vi "КЛАВИАТУРА ПОЛНАЯSMALL.vi"(8 "ВХОД ИЗМЕНЕНИЕ":string, 11 "ВХОД СТАРОЕ":string) -> (3 "ВЫХОД РЕЗУЛЬТАТ":string)   [LabVIEW 2016, in "Library.lvlib"]
uses:
  Granule-2000AT/PC/Library.lvlib
panel:
  in  "+":bool
  in  "УДАЛИТЬ":bool
  in  "ОТМЕНА":bool
  in  "ВВОД":bool
  in  "0":bool
  in  "3":bool
  in  "2":bool
  in  "1":bool
  in  "6":bool
  in  "5":bool
  in  "4":bool
  in  "8":bool
  in  "9":bool
  in  "7":bool
  in  "ПРОБЕЛ":bool
  in  "/":bool
  in  "Ю":bool
  in  "Б":bool
  in  "Ь":bool
  in  "Т":bool
  in  "И":bool
  in  "М":bool
  in  "С":bool
  in  "Ч":bool
  in  "Я":bool
  in  "\\":bool
  in  "Э":bool
  in  "Ж":bool
  in  "Д":bool
  in  "Л":bool
  in  "О":bool
  in  "Р":bool
  in  "П":bool
  in  "А":bool
  in  "В":bool
  in  "Ы":bool
  in  "Ф":bool
  in  "Ъ":bool
  in  "Х":bool
  in  "З":bool
  in  "Щ":bool
  in  "Ш":bool
  in  "Г":bool
  in  "Н":bool
  in  "Е":bool
  in  "К":bool
  in  "У":bool
  in  "Ц":bool
  in  "Й":bool
  in  "-":bool
  in  "RU":bool
  in  "=":bool
  in  ")":bool
  in  "(":bool
  in  "*":bool
  in  "?":bool
  in  ":":bool
  in  "%":bool
  in  ";":bool
  in  "№":bool
  in  "\"":bool
  in  "!":bool
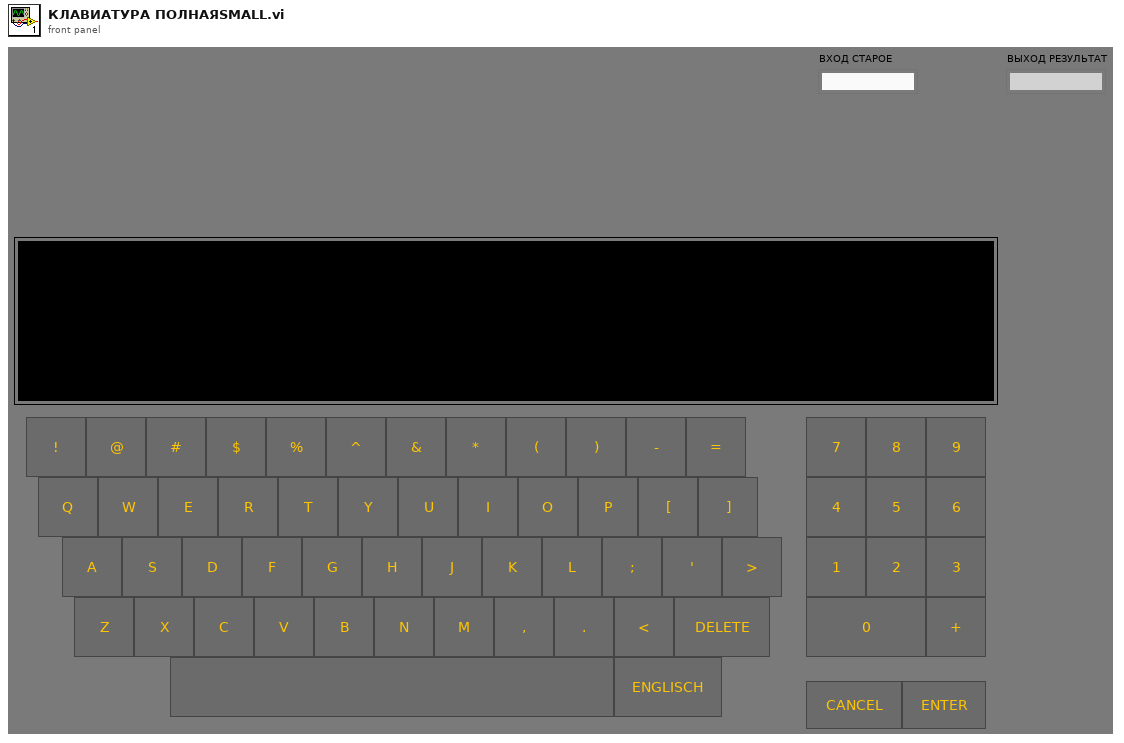
[diagram p1: front panel]
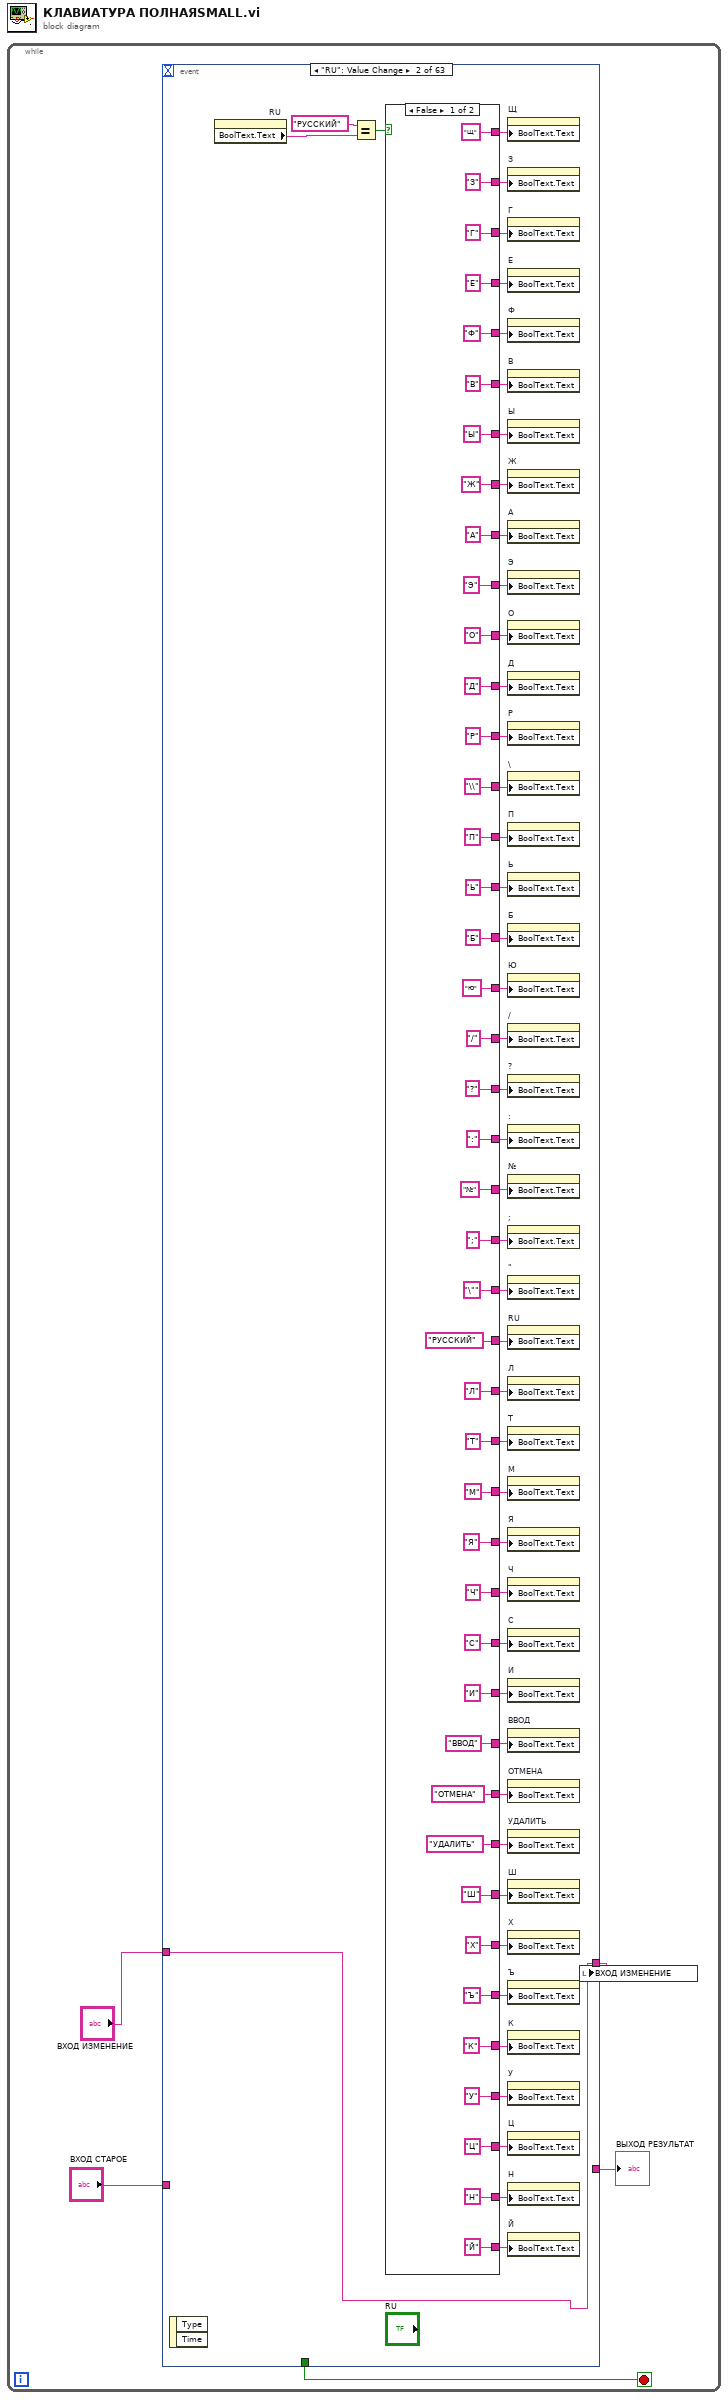
[diagram p0: block diagram]
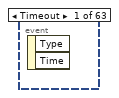
[diagram p2: hidden frame]
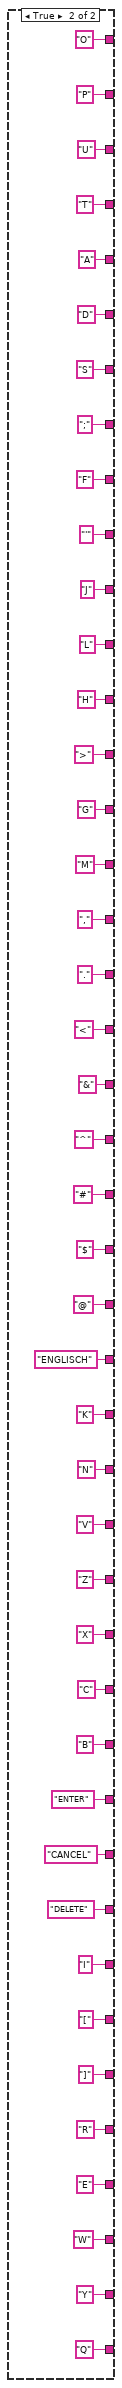
[diagram p3: hidden frame]
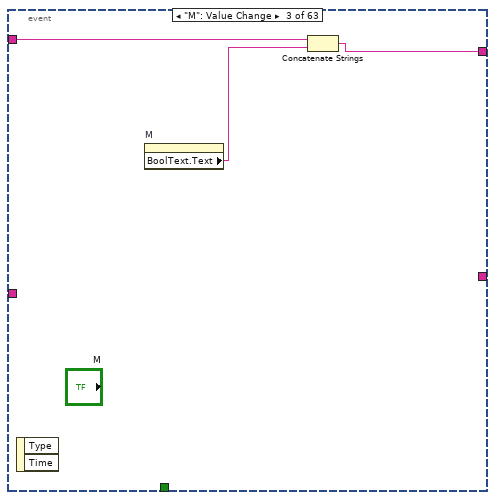
[diagram p4: hidden frame]
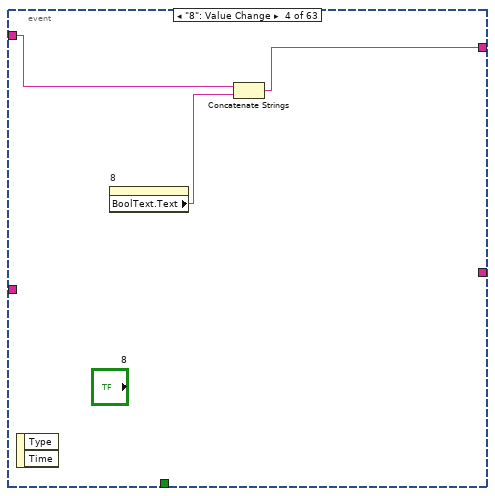
[diagram p5: hidden frame]
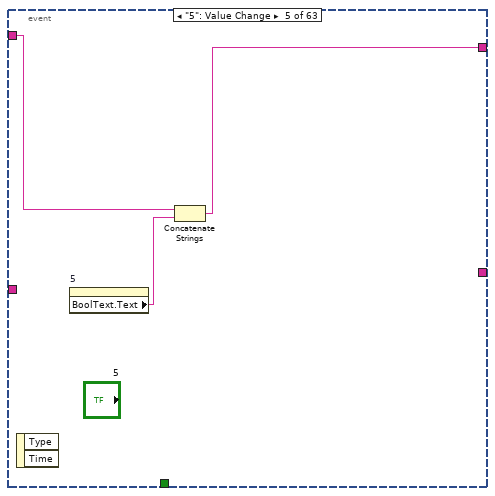
[diagram p6: hidden frame]
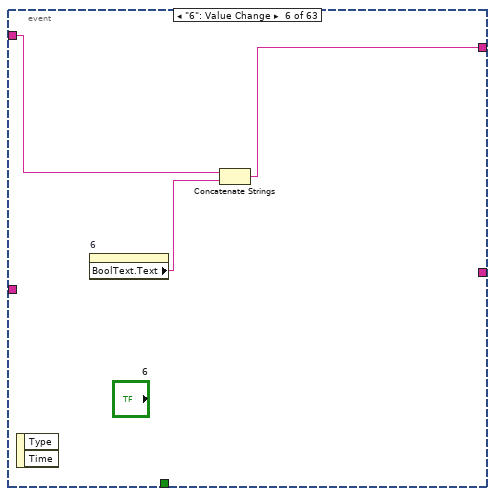
[diagram p7: hidden frame]
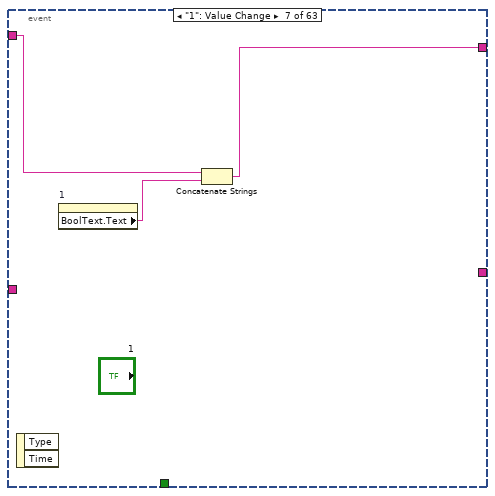
[diagram p8: hidden frame]
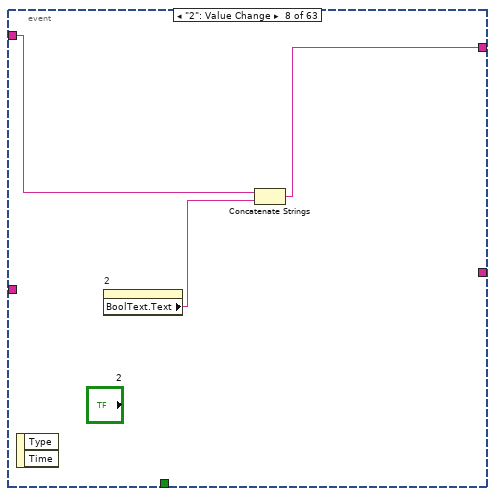
[diagram p9: hidden frame]
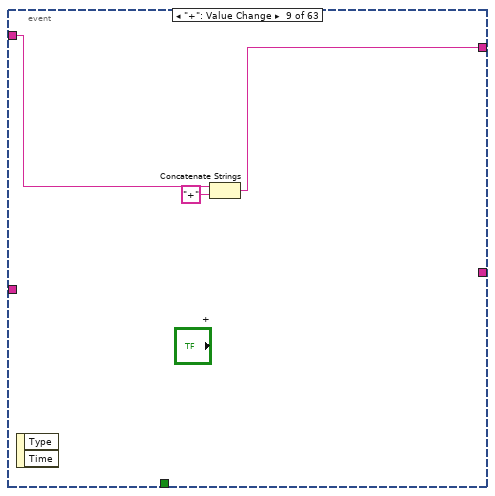
[diagram p10: hidden frame]
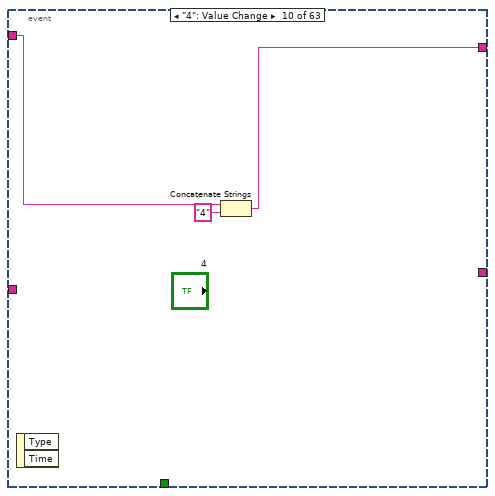
[diagram p11: hidden frame]
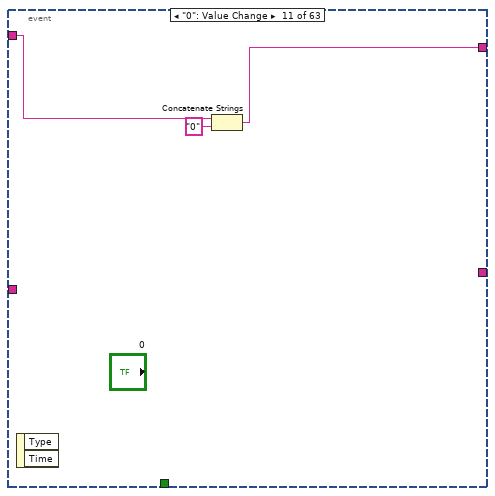
[diagram p12: hidden frame]
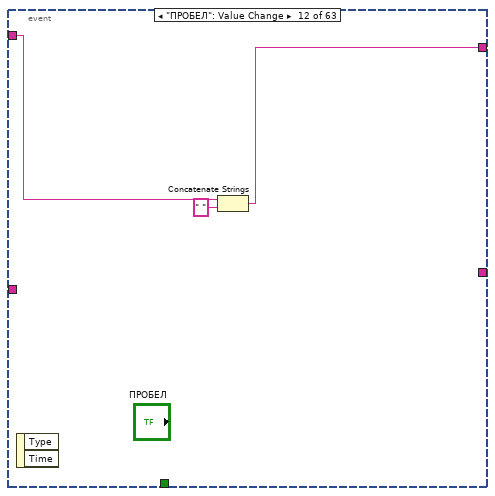
[diagram p13: hidden frame]
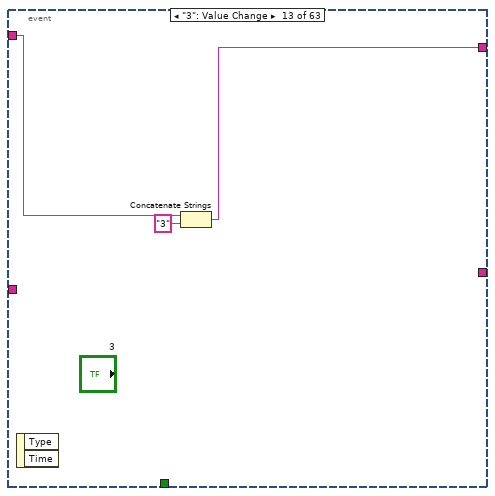
[diagram p14: hidden frame]
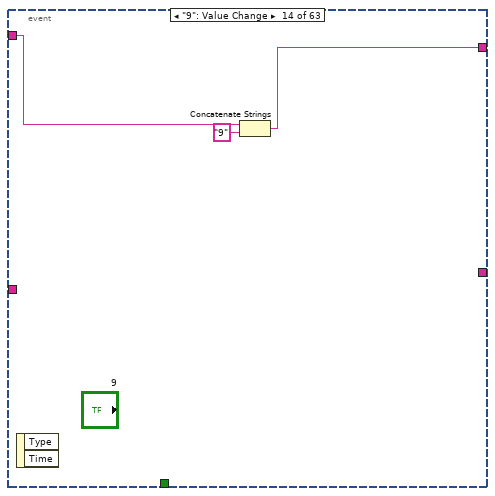
[diagram p15: hidden frame]
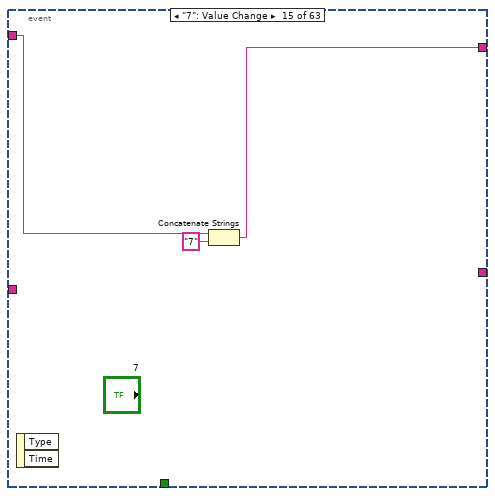
[diagram p16: hidden frame]
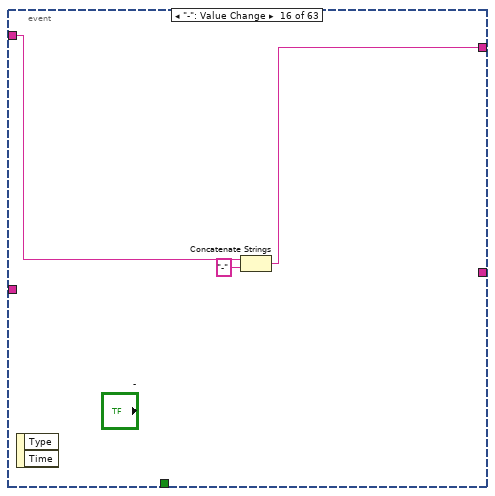
[diagram p17: hidden frame]
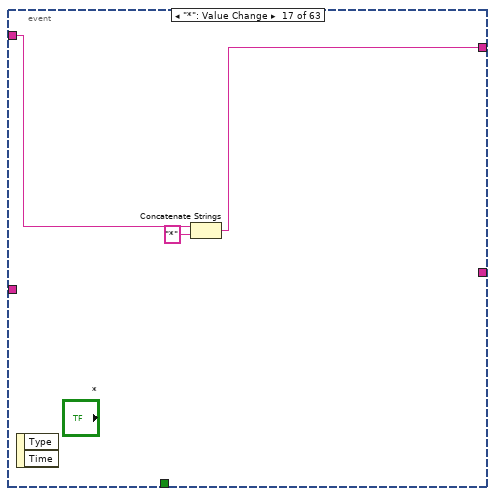
[diagram p18: hidden frame]
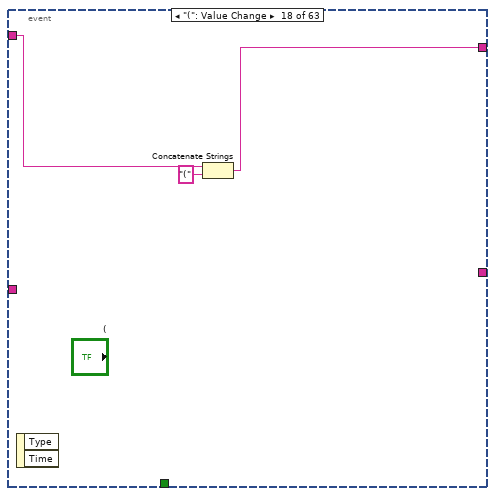
[diagram p19: hidden frame]
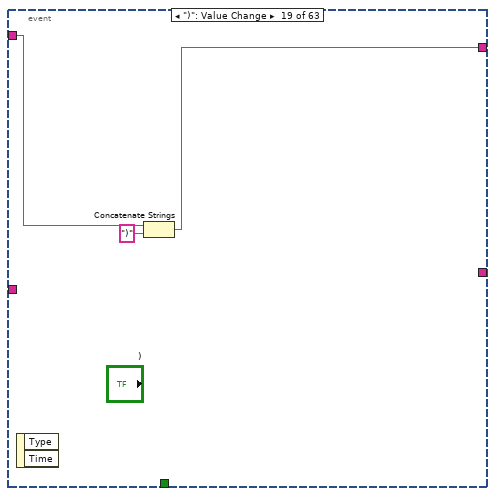
[diagram p20: hidden frame]
diagram:
  n1 = while {
    stop <- w1 stop-if-true
    n2 = event shown="[1] \"RU\": Value Change" {
      selector: _ -> [_ _ _ _ _ _ _ _ _ _ _ _ _ _ _ _ _ _ _ _ _ _ _ _ _ _ _ _ _ _ _ _ _ _ _ _ _ _ _ _ _ _ _ _ _ _ _ _ _ _ _ _ _ _ _ _ _ _ _ _ _ _ _]
      dyn-events: _ -> [_ _ _ _ _ _ _ _ _ _ _ _ _ _ _ _ _ _ _ _ _ _ _ _ _ _ _ _ _ _ _ _ _ _ _ _ _ _ _ _ _ _ _ _ _ _ _ _ _ _ _ _ _ _ _ _ _ _ _ _ _ _ _]
      timeout: _ -> [_ _ _ _ _ _ _ _ _ _ _ _ _ _ _ _ _ _ _ _ _ _ _ _ _ _ _ _ _ _ _ _ _ _ _ _ _ _ _ _ _ _ _ _ _ _ _ _ _ _ _ _ _ _ _ _ _ _ _ _ _ _ _]
      tunnel: "ВХОД ИЗМЕНЕНИЕ" -> [_ w6 w141 w144 w147 w149 w153 w156 w159 w162 w165 w168 w171 w174 w177 w180 w183 w186 w189 w192 w199 w205 w207 w211 w214 w217 w219 w222 w225 w229 w232 w234 w238 w240 w244 w246 w249 w252 w256 w258 w262 w265 w268 w270 w273 w277 w280 w283 w286 w289 w292 w295 w297 w300 w304 w307 w310 w313 w315 w318 w322 w323 w327]
      tunnel: [_ w6 w139 w143 w146 w148 w151 w155 w157 w160 w163 w167 w169 w172 w175 w178 w181 w184 w188 w190 w198 w203 w206 w209 w212 w215 w218 w221 w224 w227 w230 w233 w236 w239 w243 w245 w248 w251 w254 w257 w260 w264 w266 w269 w272 w275 w278 w281 w284 w287 w290 w293 w296 w299 w302 w305 w308 w311 w314 w317 w321 w323 w327] -> w4
      tunnel: [_ _ _ _ _ _ _ _ _ _ _ _ _ _ _ _ _ _ _ _ _ _ _ _ _ _ _ _ _ _ _ _ _ _ _ _ _ _ _ _ _ _ _ _ _ _ _ _ _ _ _ _ _ _ _ _ _ _ _ _ _ w325 w327] -> w3
      tunnel: "ВХОД СТАРОЕ" -> [_ _ _ _ _ _ _ _ _ _ _ _ _ _ _ _ _ _ _ _ _ _ _ _ _ _ _ _ _ _ _ _ _ _ _ _ _ _ _ _ _ _ _ _ _ _ _ _ _ _ _ _ _ _ _ _ _ _ _ _ _ w325 _]
      tunnel: [_ _ _ _ _ _ _ _ _ _ _ _ _ _ _ _ _ _ _ _ _ _ _ _ _ _ _ _ _ _ _ _ _ _ _ _ _ _ _ _ _ _ _ _ _ _ _ _ _ _ _ _ _ _ _ _ _ _ _ _ _ "ОТМЕНА" "ВВОД"] -> w1
      event Timeout {
        n3 = event-data() -> ()  [unwired: 1 in, 2 out]
      }
      event "RU": Value Change {
        n4 = event-data() -> ()  [unwired: 1 in, 2 out]
        n5 = property on="RU" class="Bool"() -> ("BoolText.Text"=w51:string)  [unwired: 2 in, 2 out]
        n6 = Equal?(x="РУССКИЙ", y=w51) -> (x = y?=w52:bool)
        n7 = case shown="False" w52 {
          tunnel: ["РУССКИЙ" ("Boolean Text.Text") "ENGLISCH" ("Boolean Text.Text")] -> w49
          tunnel: ["\"" ("Boolean Text.Text") "@" ("Boolean Text.Text")] -> w48
          tunnel: [";" ("Boolean Text.Text") "$" ("Boolean Text.Text")] -> w47
          tunnel: ["№" ("Boolean Text.Text") "#" ("Boolean Text.Text")] -> w46
          tunnel: [":" ("Boolean Text.Text") "^" ("Boolean Text.Text")] -> w45
          tunnel: ["?" ("Boolean Text.Text") "&" ("Boolean Text.Text")] -> w44
          tunnel: ["Й" ("Boolean Text.Text") "Q" ("Boolean Text.Text")] -> w43
          tunnel: ["Н" ("Boolean Text.Text") "Y" ("Boolean Text.Text")] -> w42
          tunnel: ["Ц" ("Boolean Text.Text") "W" ("Boolean Text.Text")] -> w41
          tunnel: ["У" ("Boolean Text.Text") "E" ("Boolean Text.Text")] -> w40
          tunnel: ["К" ("Boolean Text.Text") "R" ("Boolean Text.Text")] -> w39
          tunnel: ["Ъ" ("Boolean Text.Text") "]" ("Boolean Text.Text")] -> w38
          tunnel: ["Х" ("Boolean Text.Text") "[" ("Boolean Text.Text")] -> w37
          tunnel: ["Ш" ("Boolean Text.Text") "I" ("Boolean Text.Text")] -> w36
          tunnel: ["Щ" ("Boolean Text.Text") "O" ("Boolean Text.Text")] -> w35
          tunnel: ["З" ("Boolean Text.Text") "P" ("Boolean Text.Text")] -> w34
          tunnel: ["Г" ("Boolean Text.Text") "U" ("Boolean Text.Text")] -> w33
          tunnel: ["Е" ("Boolean Text.Text") "T" ("Boolean Text.Text")] -> w32
          tunnel: ["Ф" ("Boolean Text.Text") "A" ("Boolean Text.Text")] -> w31
          tunnel: ["В" ("Boolean Text.Text") "D" ("Boolean Text.Text")] -> w30
          tunnel: ["Ы" ("Boolean Text.Text") "S" ("Boolean Text.Text")] -> w29
          tunnel: ["Ж" ("Boolean Text.Text") ";" ("Boolean Text.Text")] -> w28
          tunnel: ["А" ("Boolean Text.Text") "F" ("Boolean Text.Text")] -> w27
          tunnel: ["Э" ("Boolean Text.Text") "'" ("Boolean Text.Text")] -> w26
          tunnel: ["О" ("Boolean Text.Text") "J" ("Boolean Text.Text")] -> w25
          tunnel: ["Д" ("Boolean Text.Text") "L" ("Boolean Text.Text")] -> w24
          tunnel: ["Р" ("Boolean Text.Text") "H" ("Boolean Text.Text")] -> w23
          tunnel: ["\\" ("Boolean Text.Text") ">" ("Boolean Text.Text")] -> w22
          tunnel: ["П" ("Boolean Text.Text") "G" ("Boolean Text.Text")] -> w21
          tunnel: ["Л" ("Boolean Text.Text") "K" ("Boolean Text.Text")] -> w20
          tunnel: ["ОТМЕНА" ("Boolean Text.Text") "CANCEL" ("Boolean Text.Text")] -> w19
          tunnel: ["ВВОД" ("Boolean Text.Text") "ENTER" ("Boolean Text.Text")] -> w18
          tunnel: ["УДАЛИТЬ" ("Boolean Text.Text") "DELETE" ("Boolean Text.Text")] -> w17
          tunnel: ["Я" ("Boolean Text.Text") "Z" ("Boolean Text.Text")] -> w16
          tunnel: ["Ч" ("Boolean Text.Text") "X" ("Boolean Text.Text")] -> w15
          tunnel: ["С" ("Boolean Text.Text") "C" ("Boolean Text.Text")] -> w14
          tunnel: ["М" ("Boolean Text.Text") "V" ("Boolean Text.Text")] -> w13
          tunnel: ["И" ("Boolean Text.Text") "B" ("Boolean Text.Text")] -> w12
          tunnel: ["Т" ("Boolean Text.Text") "N" ("Boolean Text.Text")] -> w11
          tunnel: ["Ь" ("Boolean Text.Text") "M" ("Boolean Text.Text")] -> w10
          tunnel: ["Б" ("Boolean Text.Text") "," ("Boolean Text.Text")] -> w9
          tunnel: ["Ю" ("Boolean Text.Text") "." ("Boolean Text.Text")] -> w8
          tunnel: ["/" ("Boolean Text.Text") "<" ("Boolean Text.Text")] -> w7
          frame False {
          }
          frame True {
          }
        }
        n8 = property on="Щ" class="Bool"("BoolText.Text"=w35) -> ()  [unwired: 2 in, 2 out]
        n9 = property on="З" class="Bool"("BoolText.Text"=w34) -> ()  [unwired: 2 in, 2 out]
        n10 = property on="Г" class="Bool"("BoolText.Text"=w33) -> ()  [unwired: 2 in, 2 out]
        n11 = property on="Е" class="Bool"("BoolText.Text"=w32) -> ()  [unwired: 2 in, 2 out]
        n12 = property on="Ф" class="Bool"("BoolText.Text"=w31) -> ()  [unwired: 2 in, 2 out]
        n13 = property on="В" class="Bool"("BoolText.Text"=w30) -> ()  [unwired: 2 in, 2 out]
        n14 = property on="Ы" class="Bool"("BoolText.Text"=w29) -> ()  [unwired: 2 in, 2 out]
        n15 = property on="Ж" class="Bool"("BoolText.Text"=w28) -> ()  [unwired: 2 in, 2 out]
        n16 = property on="А" class="Bool"("BoolText.Text"=w27) -> ()  [unwired: 2 in, 2 out]
        n17 = property on="Э" class="Bool"("BoolText.Text"=w26) -> ()  [unwired: 2 in, 2 out]
        n18 = property on="О" class="Bool"("BoolText.Text"=w25) -> ()  [unwired: 2 in, 2 out]
        n19 = property on="Д" class="Bool"("BoolText.Text"=w24) -> ()  [unwired: 2 in, 2 out]
        n20 = property on="Р" class="Bool"("BoolText.Text"=w23) -> ()  [unwired: 2 in, 2 out]
        n21 = property on="\\" class="Bool"("BoolText.Text"=w22) -> ()  [unwired: 2 in, 2 out]
        n22 = property on="П" class="Bool"("BoolText.Text"=w21) -> ()  [unwired: 2 in, 2 out]
        n23 = property on="Ь" class="Bool"("BoolText.Text"=w10) -> ()  [unwired: 2 in, 2 out]
        n24 = property on="Б" class="Bool"("BoolText.Text"=w9) -> ()  [unwired: 2 in, 2 out]
        n25 = property on="Ю" class="Bool"("BoolText.Text"=w8) -> ()  [unwired: 2 in, 2 out]
        n26 = property on="/" class="Bool"("BoolText.Text"=w7) -> ()  [unwired: 2 in, 2 out]
        n27 = property on="?" class="Bool"("BoolText.Text"=w44) -> ()  [unwired: 2 in, 2 out]
        n28 = property on=":" class="Bool"("BoolText.Text"=w45) -> ()  [unwired: 2 in, 2 out]
        n29 = property on="№" class="Bool"("BoolText.Text"=w46) -> ()  [unwired: 2 in, 2 out]
        n30 = property on=";" class="Bool"("BoolText.Text"=w47) -> ()  [unwired: 2 in, 2 out]
        n31 = property on="\"" class="Bool"("BoolText.Text"=w48) -> ()  [unwired: 2 in, 2 out]
        n32 = property on="RU" class="Bool"("BoolText.Text"=w49) -> ()  [unwired: 2 in, 2 out]
        n33 = property on="Л" class="Bool"("BoolText.Text"=w20) -> ()  [unwired: 2 in, 2 out]
        n34 = property on="Т" class="Bool"("BoolText.Text"=w11) -> ()  [unwired: 2 in, 2 out]
        n35 = property on="М" class="Bool"("BoolText.Text"=w13) -> ()  [unwired: 2 in, 2 out]
        n36 = property on="Я" class="Bool"("BoolText.Text"=w16) -> ()  [unwired: 2 in, 2 out]
        n37 = property on="Ч" class="Bool"("BoolText.Text"=w15) -> ()  [unwired: 2 in, 2 out]
        n38 = property on="С" class="Bool"("BoolText.Text"=w14) -> ()  [unwired: 2 in, 2 out]
        n39 = property on="И" class="Bool"("BoolText.Text"=w12) -> ()  [unwired: 2 in, 2 out]
        n40 = property on="ВВОД" class="Bool"("BoolText.Text"=w18) -> ()  [unwired: 2 in, 2 out]
        n41 = property on="ОТМЕНА" class="Bool"("BoolText.Text"=w19) -> ()  [unwired: 2 in, 2 out]
        n42 = property on="УДАЛИТЬ" class="Bool"("BoolText.Text"=w17) -> ()  [unwired: 2 in, 2 out]
        n43 = property on="Ш" class="Bool"("BoolText.Text"=w36) -> ()  [unwired: 2 in, 2 out]
        n44 = property on="Х" class="Bool"("BoolText.Text"=w37) -> ()  [unwired: 2 in, 2 out]
        n45 = property on="Ъ" class="Bool"("BoolText.Text"=w38) -> ()  [unwired: 2 in, 2 out]
        n46 = property on="К" class="Bool"("BoolText.Text"=w39) -> ()  [unwired: 2 in, 2 out]
        n47 = property on="У" class="Bool"("BoolText.Text"=w40) -> ()  [unwired: 2 in, 2 out]
        n48 = property on="Ц" class="Bool"("BoolText.Text"=w41) -> ()  [unwired: 2 in, 2 out]
        n49 = property on="Н" class="Bool"("BoolText.Text"=w42) -> ()  [unwired: 2 in, 2 out]
        n50 = property on="Й" class="Bool"("BoolText.Text"=w43) -> ()  [unwired: 2 in, 2 out]
      }
      event "М": Value Change {
        n51 = event-data() -> ()  [unwired: 1 in, 2 out]
        n52 = property on="М" class="Bool"() -> ("BoolText.Text"=w140:string)  [unwired: 2 in, 2 out]
        n53 = Concatenate Strings(w141, w140) -> (w139:string)
      }
      event "8": Value Change {
        n54 = event-data() -> ()  [unwired: 1 in, 2 out]
        n55 = property on="8" class="Bool"() -> ("BoolText.Text"=w142:string)  [unwired: 2 in, 2 out]
        n56 = Concatenate Strings(w144, w142) -> (w143:string)
      }
      event "5": Value Change {
        n57 = event-data() -> ()  [unwired: 1 in, 2 out]
        n58 = property on="5" class="Bool"() -> ("BoolText.Text"=w145:string)  [unwired: 2 in, 2 out]
        n59 = Concatenate Strings(w147, w145) -> (w146:string)
      }
      event "6": Value Change {
        n60 = event-data() -> ()  [unwired: 1 in, 2 out]
        n61 = property on="6" class="Bool"() -> ("BoolText.Text"=w150:string)  [unwired: 2 in, 2 out]
        n62 = Concatenate Strings(w149, w150) -> (w148:string)
      }
      event "1": Value Change {
        n63 = event-data() -> ()  [unwired: 1 in, 2 out]
        n64 = property on="1" class="Bool"() -> ("BoolText.Text"=w152:string)  [unwired: 2 in, 2 out]
        n65 = Concatenate Strings(w153, w152) -> (w151:string)
      }
      event "2": Value Change {
        n66 = event-data() -> ()  [unwired: 1 in, 2 out]
        n67 = property on="2" class="Bool"() -> ("BoolText.Text"=w154:string)  [unwired: 2 in, 2 out]
        n68 = Concatenate Strings(w156, w154) -> (w155:string)
      }
      event "+": Value Change {
        n69 = event-data() -> ()  [unwired: 1 in, 2 out]
        n70 = Concatenate Strings(w159, "+" ("string")) -> (w157:string)
      }
      event "4": Value Change {
        n71 = event-data() -> ()  [unwired: 1 in, 2 out]
        n72 = Concatenate Strings(w162, "4" ("string")) -> (w160:string)
      }
      event "0": Value Change {
        n73 = event-data() -> ()  [unwired: 1 in, 2 out]
        n74 = Concatenate Strings(w165, "0" ("string")) -> (w163:string)
      }
      event "ПРОБЕЛ": Value Change {
        n75 = event-data() -> ()  [unwired: 1 in, 2 out]
        n76 = Concatenate Strings(w168, " " ("string")) -> (w167:string)
      }
      event "3": Value Change {
        n77 = event-data() -> ()  [unwired: 1 in, 2 out]
        n78 = Concatenate Strings(w171, "3" ("string")) -> (w169:string)
      }
      event "9": Value Change {
        n79 = event-data() -> ()  [unwired: 1 in, 2 out]
        n80 = Concatenate Strings(w174, "9" ("string")) -> (w172:string)
      }
      event "7": Value Change {
        n81 = event-data() -> ()  [unwired: 1 in, 2 out]
        n82 = Concatenate Strings(w177, "7" ("string")) -> (w175:string)
      }
      event "-": Value Change {
        n83 = event-data() -> ()  [unwired: 1 in, 2 out]
        n84 = Concatenate Strings(w180, "-" ("string")) -> (w178:string)
      }
      event "*": Value Change {
        n85 = event-data() -> ()  [unwired: 1 in, 2 out]
        n86 = Concatenate Strings(w183, "*" ("string")) -> (w181:string)
      }
      event "(": Value Change {
        n87 = event-data() -> ()  [unwired: 1 in, 2 out]
        n88 = Concatenate Strings(w186, "(" ("string")) -> (w184:string)
      }
      event ")": Value Change {
        n89 = event-data() -> ()  [unwired: 1 in, 2 out]
        n90 = Concatenate Strings(w189, ")" ("string")) -> (w188:string)
      }
      event "=": Value Change {
        n91 = event-data() -> ()  [unwired: 1 in, 2 out]
        n92 = Concatenate Strings(w192, "=" ("string")) -> (w190:string)
      }
      event "УДАЛИТЬ": Value Change {
        n93 = event-data() -> ()  [unwired: 1 in, 2 out]
        n94 = String Length(string=w199) -> (length=w196:i32)
        n95 = Less Or Equal?(x=w196, y=0) -> (x <= y?=w194:bool)
        n96 = Not(x=w194) -> (.not. x?=w193:bool)
        n97 = case shown="False" w193 {
          tunnel: w196 -> [w200 w202]
          tunnel: [w200 w201] -> w195
          frame False {
          }
          frame True {
            n98 = Decrement(x=w202) -> (x-1=w201:i32)
          }
        }
        n99 = String Subset(string=w199, length (rest)=w195) -> (substring=w198:string)  [unwired: 1 in]
      }
      event "А": Value Change {
        n100 = event-data() -> ()  [unwired: 1 in, 2 out]
        n101 = property on="А" class="Bool"() -> ("BoolText.Text"=w204:string)  [unwired: 2 in, 2 out]
        n102 = Concatenate Strings(w205, w204) -> (w203:string)
      }
      event "Л": Value Change {
        n103 = event-data() -> ()  [unwired: 1 in, 2 out]
        n104 = property on="Л" class="Bool"() -> ("BoolText.Text"=w208:string)  [unwired: 2 in, 2 out]
        n105 = Concatenate Strings(w207, w208) -> (w206:string)
      }
      event "Й": Value Change {
        n106 = event-data() -> ()  [unwired: 1 in, 2 out]
        n107 = property on="Й" class="Bool"() -> ("BoolText.Text"=w210:string)  [unwired: 2 in, 2 out]
        n108 = Concatenate Strings(w211, w210) -> (w209:string)
      }
      event "?": Value Change {
        n109 = event-data() -> ()  [unwired: 1 in, 2 out]
        n110 = property on="?" class="Bool"() -> ("BoolText.Text"=w213:string)  [unwired: 2 in, 2 out]
        n111 = Concatenate Strings(w214, w213) -> (w212:string)
      }
      event "\"": Value Change {
        n112 = event-data() -> ()  [unwired: 1 in, 2 out]
        n113 = property on="\"" class="Bool"() -> ("BoolText.Text"=w216:string)  [unwired: 2 in, 2 out]
        n114 = Concatenate Strings(w217, w216) -> (w215:string)
      }
      event "%": Value Change {
        n115 = event-data() -> ()  [unwired: 1 in, 2 out]
        n116 = property on="%" class="Bool"() -> ("BoolText.Text"=w220:string)  [unwired: 2 in, 2 out]
        n117 = Concatenate Strings(w219, w220) -> (w218:string)
      }
      event "!": Value Change {
        n118 = event-data() -> ()  [unwired: 1 in, 2 out]
        n119 = property on="!" class="Bool"() -> ("BoolText.Text"=w223:string)  [unwired: 2 in, 2 out]
        n120 = Concatenate Strings(w222, w223) -> (w221:string)
      }
      event ";": Value Change {
        n121 = event-data() -> ()  [unwired: 1 in, 2 out]
        n122 = property on=";" class="Bool"() -> ("BoolText.Text"=w226:string)  [unwired: 2 in, 2 out]
        n123 = Concatenate Strings(w225, w226) -> (w224:string)
      }
      event "№": Value Change {
        n124 = event-data() -> ()  [unwired: 1 in, 2 out]
        n125 = property on="№" class="Bool"() -> ("BoolText.Text"=w228:string)  [unwired: 2 in, 2 out]
        n126 = Concatenate Strings(w229, w228) -> (w227:string)
      }
      event "\\": Value Change {
        n127 = event-data() -> ()  [unwired: 1 in, 2 out]
        n128 = property on="\\" class="Bool"() -> ("BoolText.Text"=w231:string)  [unwired: 2 in, 2 out]
        n129 = Concatenate Strings(w232, w231) -> (w230:string)
      }
      event "/": Value Change {
        n130 = event-data() -> ()  [unwired: 1 in, 2 out]
        n131 = property on="/" class="Bool"() -> ("BoolText.Text"=w235:string)  [unwired: 2 in, 2 out]
        n132 = Concatenate Strings(w234, w235) -> (w233:string)
      }
      event ":": Value Change {
        n133 = event-data() -> ()  [unwired: 1 in, 2 out]
        n134 = property on=":" class="Bool"() -> ("BoolText.Text"=w237:string)  [unwired: 2 in, 2 out]
        n135 = Concatenate Strings(w238, w237) -> (w236:string)
      }
      event "Ь": Value Change {
        n136 = event-data() -> ()  [unwired: 1 in, 2 out]
        n137 = property on="Ь" class="Bool"() -> ("BoolText.Text"=w241:string)  [unwired: 2 in, 2 out]
        n138 = Concatenate Strings(w240, w241) -> (w239:string)
      }
      event "Р": Value Change {
        n139 = event-data() -> ()  [unwired: 1 in, 2 out]
        n140 = property on="Р" class="Bool"() -> ("BoolText.Text"=w242:string)  [unwired: 2 in, 2 out]
        n141 = Concatenate Strings(w244, w242) -> (w243:string)
      }
      event "Х": Value Change {
        n142 = event-data() -> ()  [unwired: 1 in, 2 out]
        n143 = property on="Х" class="Bool"() -> ("BoolText.Text"=w247:string)  [unwired: 2 in, 2 out]
        n144 = Concatenate Strings(w246, w247) -> (w245:string)
      }
      event "Т": Value Change {
        n145 = event-data() -> ()  [unwired: 1 in, 2 out]
        n146 = property on="Т" class="Bool"() -> ("BoolText.Text"=w250:string)  [unwired: 2 in, 2 out]
        n147 = Concatenate Strings(w249, w250) -> (w248:string)
      }
      event "Б": Value Change {
        n148 = event-data() -> ()  [unwired: 1 in, 2 out]
        n149 = property on="Б" class="Bool"() -> ("BoolText.Text"=w253:string)  [unwired: 2 in, 2 out]
        n150 = Concatenate Strings(w252, w253) -> (w251:string)
      }
      event "Д": Value Change {
        n151 = event-data() -> ()  [unwired: 1 in, 2 out]
        n152 = property on="Д" class="Bool"() -> ("BoolText.Text"=w255:string)  [unwired: 2 in, 2 out]
        n153 = Concatenate Strings(w256, w255) -> (w254:string)
      }
      event "Щ": Value Change {
        n154 = event-data() -> ()  [unwired: 1 in, 2 out]
        n155 = property on="Щ" class="Bool"() -> ("BoolText.Text"=w259:string)  [unwired: 2 in, 2 out]
        n156 = Concatenate Strings(w258, w259) -> (w257:string)
      }
      event "Е": Value Change {
        n157 = event-data() -> ()  [unwired: 1 in, 2 out]
        n158 = property on="Е" class="Bool"() -> ("BoolText.Text"=w261:string)  [unwired: 2 in, 2 out]
        n159 = Concatenate Strings(w262, w261) -> (w260:string)
      }
      event "Ъ": Value Change {
        n160 = event-data() -> ()  [unwired: 1 in, 2 out]
        n161 = property on="Ъ" class="Bool"() -> ("BoolText.Text"=w263:string)  [unwired: 2 in, 2 out]
        n162 = Concatenate Strings(w265, w263) -> (w264:string)
      }
      event "В": Value Change {
        n163 = event-data() -> ()  [unwired: 1 in, 2 out]
        n164 = property on="В" class="Bool"() -> ("BoolText.Text"=w267:string)  [unwired: 2 in, 2 out]
        n165 = Concatenate Strings(w268, w267) -> (w266:string)
      }
      event "Ы": Value Change {
        n166 = event-data() -> ()  [unwired: 1 in, 2 out]
        n167 = property on="Ы" class="Bool"() -> ("BoolText.Text"=w271:string)  [unwired: 2 in, 2 out]
        n168 = Concatenate Strings(w270, w271) -> (w269:string)
      }
      event "Ф": Value Change {
        n169 = event-data() -> ()  [unwired: 1 in, 2 out]
        n170 = property on="Ф" class="Bool"() -> ("BoolText.Text"=w274:string)  [unwired: 2 in, 2 out]
        n171 = Concatenate Strings(w273, w274) -> (w272:string)
      }
      event "Г": Value Change {
        n172 = event-data() -> ()  [unwired: 1 in, 2 out]
        n173 = property on="Г" class="Bool"() -> ("BoolText.Text"=w276:string)  [unwired: 2 in, 2 out]
        n174 = Concatenate Strings(w277, w276) -> (w275:string)
      }
      event "Ш": Value Change {
        n175 = event-data() -> ()  [unwired: 1 in, 2 out]
        n176 = property on="Ш" class="Bool"() -> ("BoolText.Text"=w279:string)  [unwired: 2 in, 2 out]
        n177 = Concatenate Strings(w280, w279) -> (w278:string)
      }
      event "С": Value Change {
        n178 = event-data() -> ()  [unwired: 1 in, 2 out]
        n179 = property on="С" class="Bool"() -> ("BoolText.Text"=w282:string)  [unwired: 2 in, 2 out]
        n180 = Concatenate Strings(w283, w282) -> (w281:string)
      }
      event "Ж": Value Change {
        n181 = event-data() -> ()  [unwired: 1 in, 2 out]
        n182 = property on="Ж" class="Bool"() -> ("BoolText.Text"=w285:string)  [unwired: 2 in, 2 out]
        n183 = Concatenate Strings(w286, w285) -> (w284:string)
      }
      event "П": Value Change {
        n184 = event-data() -> ()  [unwired: 1 in, 2 out]
        n185 = property on="П" class="Bool"() -> ("BoolText.Text"=w288:string)  [unwired: 2 in, 2 out]
        n186 = Concatenate Strings(w289, w288) -> (w287:string)
      }
      event "Н": Value Change {
        n187 = event-data() -> ()  [unwired: 1 in, 2 out]
        n188 = property on="Н" class="Bool"() -> ("BoolText.Text"=w291:string)  [unwired: 2 in, 2 out]
        n189 = Concatenate Strings(w292, w291) -> (w290:string)
      }
      event "З": Value Change {
        n190 = event-data() -> ()  [unwired: 1 in, 2 out]
        n191 = property on="З" class="Bool"() -> ("BoolText.Text"=w294:string)  [unwired: 2 in, 2 out]
        n192 = Concatenate Strings(w295, w294) -> (w293:string)
      }
      event "О": Value Change {
        n193 = event-data() -> ()  [unwired: 1 in, 2 out]
        n194 = property on="О" class="Bool"() -> ("BoolText.Text"=w298:string)  [unwired: 2 in, 2 out]
        n195 = Concatenate Strings(w297, w298) -> (w296:string)
      }
      event "К": Value Change {
        n196 = event-data() -> ()  [unwired: 1 in, 2 out]
        n197 = property on="К" class="Bool"() -> ("BoolText.Text"=w301:string)  [unwired: 2 in, 2 out]
        n198 = Concatenate Strings(w300, w301) -> (w299:string)
      }
      event "Ц": Value Change {
        n199 = event-data() -> ()  [unwired: 1 in, 2 out]
        n200 = property on="Ц" class="Bool"() -> ("BoolText.Text"=w303:string)  [unwired: 2 in, 2 out]
        n201 = Concatenate Strings(w304, w303) -> (w302:string)
      }
      event "Ю": Value Change {
        n202 = event-data() -> ()  [unwired: 1 in, 2 out]
        n203 = property on="Ю" class="Bool"() -> ("BoolText.Text"=w306:string)  [unwired: 2 in, 2 out]
        n204 = Concatenate Strings(w307, w306) -> (w305:string)
      }
      event "Э": Value Change {
        n205 = event-data() -> ()  [unwired: 1 in, 2 out]
        n206 = property on="Э" class="Bool"() -> ("BoolText.Text"=w309:string)  [unwired: 2 in, 2 out]
        n207 = Concatenate Strings(w310, w309) -> (w308:string)
      }
      event "У": Value Change {
        n208 = event-data() -> ()  [unwired: 1 in, 2 out]
        n209 = property on="У" class="Bool"() -> ("BoolText.Text"=w312:string)  [unwired: 2 in, 2 out]
        n210 = Concatenate Strings(w313, w312) -> (w311:string)
      }
      event "Я": Value Change {
        n211 = event-data() -> ()  [unwired: 1 in, 2 out]
        n212 = property on="Я" class="Bool"() -> ("BoolText.Text"=w316:string)  [unwired: 2 in, 2 out]
        n213 = Concatenate Strings(w315, w316) -> (w314:string)
      }
      event "Ч": Value Change {
        n214 = event-data() -> ()  [unwired: 1 in, 2 out]
        n215 = property on="Ч" class="Bool"() -> ("BoolText.Text"=w319:string)  [unwired: 2 in, 2 out]
        n216 = Concatenate Strings(w318, w319) -> (w317:string)
      }
      event "И": Value Change {
        n217 = event-data() -> ()  [unwired: 1 in, 2 out]
        n218 = property on="И" class="Bool"() -> ("BoolText.Text"=w320:string)  [unwired: 2 in, 2 out]
        n219 = Concatenate Strings(w322, w320) -> (w321:string)
      }
      event "ОТМЕНА": Value Change {
        n220 = event-data() -> ()  [unwired: 1 in, 2 out]
      }
      event "ВВОД": Value Change {
        n221 = event-data() -> ()  [unwired: 1 in, 2 out]
      }
    }
    "ВЫХОД РЕЗУЛЬТАТ" <- w3
    n222 = local write "ВХОД ИЗМЕНЕНИЕ"(w4) -> ()
  }
